vi "Write Value.vi"(8 "error in (no error)":errorcluster, 10 "Value":variant, 11 "Tag in":refnum<class "Tag.lvclass">) -> (0 "error out":errorcluster, 3 "Tag out":refnum<class "Tag.lvclass">)   [LabVIEW 2020, in "Tag Engine Core.lvlib" / "Tag.lvclass"]
doc: "_SubVI_"
uses:
  Tag.lvclass
  Tag.lvclass/Tag.ctl
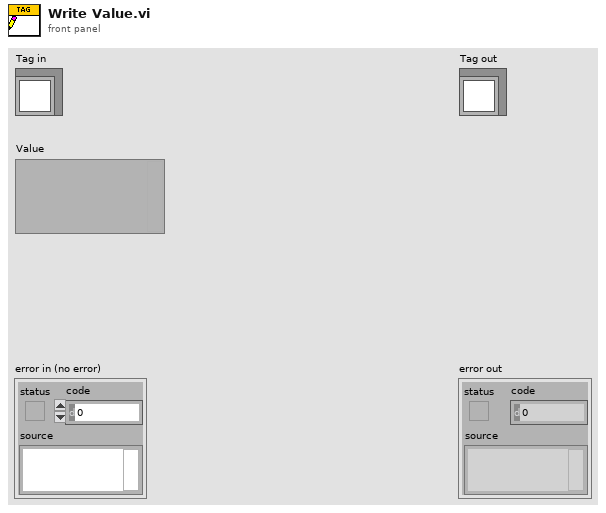
[diagram p1: front panel]
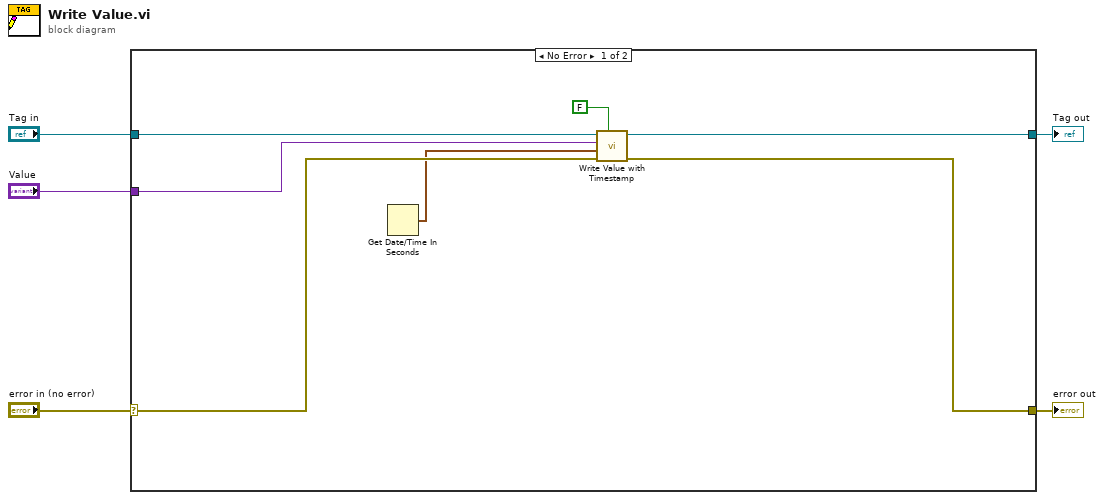
[diagram p0: block diagram]
diagram:
  n1 = case shown="No Error" "error in (no error)" {
    selector: "error in (no error)" -> [w9 w13]
    tunnel: [w8 w13] -> w4
    tunnel: [w11 w14] -> w2
    tunnel: "Tag in" -> [w12 w14]
    tunnel: "Value" -> [w10 _]
    frame No Error {
      n2 = Get Date/Time In Seconds() -> (seconds since 1Jan1904=w6:timestamp)
      n3 = call "Write Value with Timestamp.vi"("IgnoreIfEqual (F)"=FALSE, "error in (no error)"=w9, "Timestamp (now)"=w6, "Value"=w10, "Tag in"=w12) -> ("error out"=w8:errorcluster, "Tag out"=w11:refnum<class "Tag.lvclass">)  [unwired: 5 in]
    }
    frame Error {
    }
  }
  "error out" <- w4
  "Tag out" <- w2
